vi "deferPaneUpdates.vi"(8 "error in (no error)":errorcluster, 10 "Defer Updates":bool, 11 "BuildServer in":refnum<class "BuildServer.lvclass">) -> (0 "error out":errorcluster, 3 "BuildServer out":refnum<class "BuildServer.lvclass">)   [LabVIEW 2017, in "BuildServer.lvlib" / "BuildServer.lvclass"]
uses:
  BuildServer.lvclass
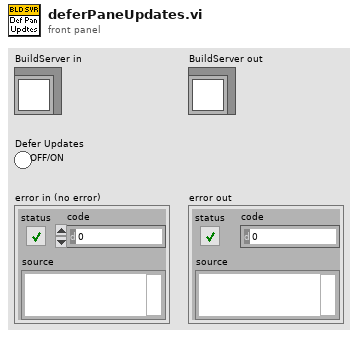
[diagram p1: front panel]
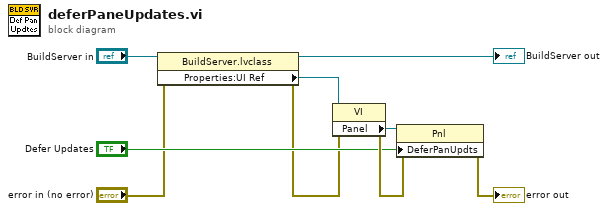
[diagram p0: block diagram]
diagram:
  n1 = property class="BuildServer.lvclass"(reference="BuildServer in", error in="error in (no error)") -> (reference out=→"BuildServer out":refnum<class "BuildServer.lvclass">, error out=w1:errorcluster, "Properties:UI Ref"=w3:refnum<vi>)
  n2 = property class="VI"(reference=w3, error in=w1) -> (error out=w8:errorcluster, "Panel"=w6:refnum<vi>)  [unwired: 1 out]
  n3 = property class="Pnl"(reference=w6, error in=w8, "DeferPanUpdts"="Defer Updates") -> (error out=→"error out":errorcluster)  [unwired: 1 out]
